vi "UTF-8 to Text (Place VI Content).vi"   [LabVIEW 2017]
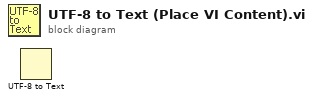
[diagram p0: block diagram]
diagram:
  n1 = UTF-8 to Text() -> ()  [unwired: 3 in, 2 out]
